vi "Global_pH.vi"() -> ()   [LabVIEW 2017]
panel:
  out "Work":bool
  out "Dangerous_Work":bool
  out "FREE":bool
  out "Temperature":dbl
  out "DO Value":dbl
  out "Minimum Alarm_TEM":bool
  out "Maximum Alarm_TEM":bool
  in  "Lower Limit_TEM":dbl
  in  "Upper Limit_TEM":dbl
  out "Minimum Alarm_DO":bool
  out "Maximum Alarm_DO":bool
  in  "Lower Limit_DO":dbl
  in  "Upper Limit_DO":dbl
  out "life of pH sensor":dbl
  in  "Stop":bool
  in  "Start":bool
  out "Minimum Alarm_pH":bool
  out "Maximum Alarm_pH":bool
  in  "Lower Limit_pH":dbl
  in  "Upper Limit_pH":dbl
  out "pH Value":dbl
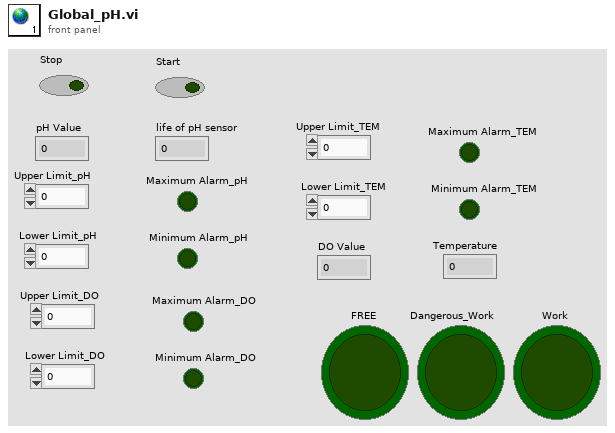
[diagram p1: front panel]
diagram:
